vi "Send dpo config.vi"(2 "Array Configuration":string[](array[string]), 3 "TCP/IP Addres":string) -> (0 "error out":errorcluster, 1 "Exit":bool)   [LabVIEW 2010]
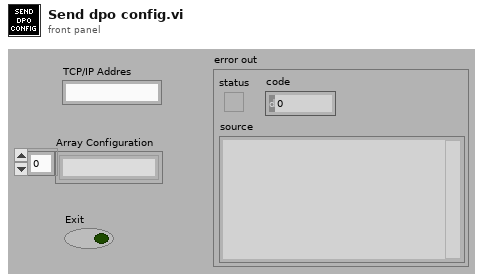
[diagram p1: front panel]
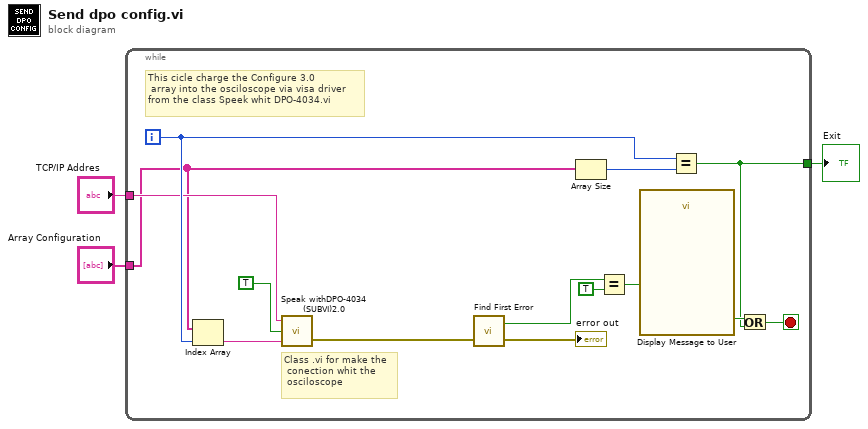
[diagram p0: block diagram]
diagram:
  n1 = while {
    tunnel: "TCP/IP Addres" -> [w8]
    tunnel: [w5] -> w3
    tunnel: "Array Configuration" -> [w4]
    i -> [w16]
    stop <- w6 stop-if-true
    # "Class .vi for make the\n conection whit the\n osciloscope"
    # "This cicle charge the Configure 3.0\n array into the osciloscope via visa driver \nfrom the class Speek whit DPO-4034.vi"
    n2 = Index Array "Index Array"(array=w4, index=w16) -> (element=w17:string)
    n3 = call "Speak withDPO-4034 (SUBVI)2.0.vi"("Send Command"=w17, "Send:  TRUE\nRecive: FALSE"=TRUE, "VISA Resource Name"=w8) -> ("error out"=w13:errorcluster)  [unwired: 1 out]
    n4 = call <vilib>:"Find First Error.vi"("error in (no error)"=w13) -> ("error out"=→"error out":errorcluster, "error?"=w9:bool)  [unwired: 3 in]
    n5 = Array Size(array=w4) -> (size(s)=w15:i32)
    n6 = Equal?(x=w9, y=TRUE) -> (x = y?=w11:bool)
    n7 = call "Display Message to User"("Enable"=w11) -> ("OK"=w7:bool)  [unwired: 9 in, 1 out]
    n8 = Equal?(x=w16, y=w15) -> (x = y?=w5:bool)
    n9 = Or(x=w7, y=w5) -> (x .or. y?=w6:bool)
  }
  "Exit" <- w3
